vi "measure_volt_ac.vi"(8 "error in (no error)":errorcluster, 9 "Resolution":dbl=-1.0 min=-2.0 format="%#_13g", 10 "Range":dbl=-1.0 min=-2.0 format="%#_13g", 11 "UI in in":T1) -> (0 "error out":errorcluster, 2 "Measurement":dbl, 3 "UI out":T1)   [LabVIEW 2017]
uses:
  ui.ctl
  classes/dc_power_supply/DC_power_supply.lvclass
  classes/report/Report.lvclass
  ui_buttons.ctl
  types/boc_type.ctl
  <instrlib>/PICOTEST M352XA/Public/Controls/Function.ctl
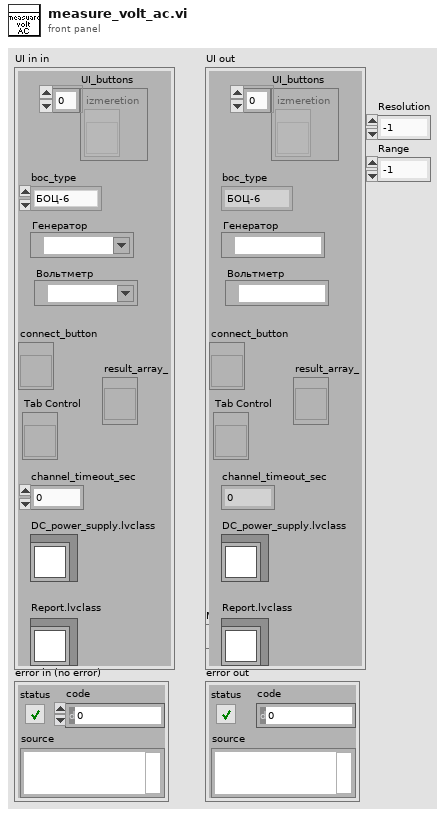
[diagram p1: front panel]
types:
  T1 = typedef "ui.ctl" = cluster{"UI_buttons":T2, "Tab Control":refnum<vi>, "connect_button":refnum<vi>, "generator":refnum<visa-resource-name>, "voltmetr":refnum<visa-resource-name>, "channel_timeout_sec":dbl, "boc_type":T3, "result_array_":refnum<vi>, "DC_power_supply.lvclass":refnum<class "DC_power_supply.lvclass">, "Report.lvclass":refnum<class "Report.lvclass">}
  T2 = typedef "ui_buttons.ctl" = refnum<vi>[]
  T3 = typedef "boc_type.ctl" = enum16{"БОЦ-6", "БОЦ-12"}
  T4 = typedef "Function.ctl" = enum16{"VOLTage:DC", "VOLTage:DC:RATio", "VOLTage:AC", "CURRent:DC", "CURRent:AC", "RESistance", "FRESistance", "FREQuency", "PERiod", "FREQuency:CURRent", "PERiod:CURRent", "CAPacitance", "CONTinuity", "DIODe", "TCOuple", "TEMPerature"}
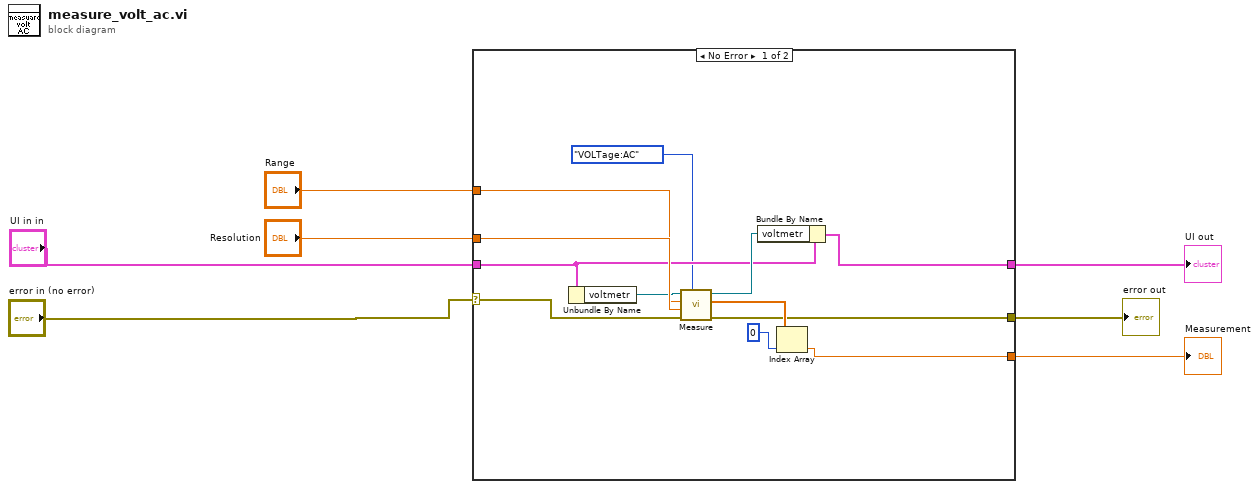
[diagram p0: block diagram]
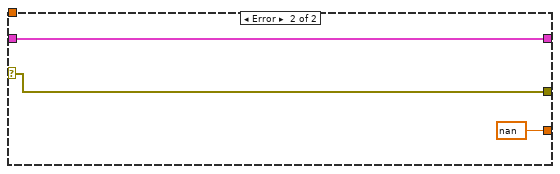
[diagram p2: hidden frame]
diagram:
  n1 = case shown="No Error" "error in (no error)" {
    selector: "error in (no error)" -> [w8 w22]
    tunnel: [w19 nan ("Measurement")] -> w7
    tunnel: "Resolution" -> [w17 _]
    tunnel: "Range" -> [w16 _]
    tunnel: [w14 w22] -> w4
    tunnel: [w12 w21] -> w3
    tunnel: "UI in in" -> [w11 w21]
    frame No Error {
      n2 = Unbundle By Name(w11) -> ("voltmetr"=w9:refnum<visa-resource-name>)
      n3 = call <instrlib>:"Measure.vi"("Function"=Function."VOLTage:AC", "error in (no error)"=w8, "Resolution"=w17, "Range"=w16, "VISA resource name"=w9) -> ("error out"=w14:errorcluster, "Measurements"=w18:dbl[], "VISA resource name out"=w13:refnum<visa-resource-name>)  [unwired: 4 in]
      n4 = Bundle By Name(cluster=w11, "voltmetr"=w13) -> (w12:T1)
      n5 = Index Array(array=w18, index=0) -> (element=w19:dbl)
    }
    frame Error {
    }
  }
  "Measurement" <- w7
  "error out" <- w4
  "UI out" <- w3
